vi "Write Type.vi"(8 "error in (no error)":errorcluster, 10 "Type":string, 11 "IV_data in":refnum<class "IV_data.lvclass">) -> (0 "error out":errorcluster, 3 "IV_data out":refnum<class "IV_data.lvclass">)   [LabVIEW 2018, in "IV_data.lvclass"]
uses:
  IV_data.lvclass
  Abstract/Data/Data2D/Data2D.lvclass
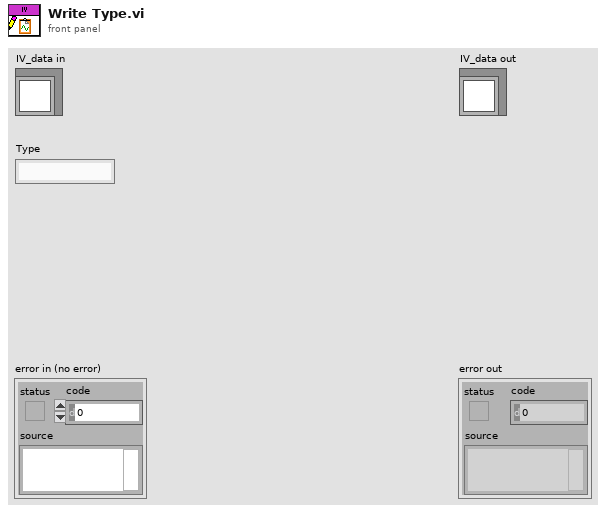
[diagram p1: front panel]
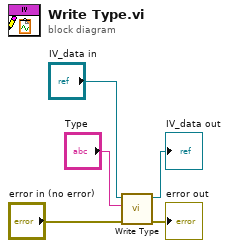
[diagram p0: block diagram]
diagram:
  n1 = call-parent "Write Type.vi"("error in (no error)"="error in (no error)", "Type"="Type", "Data2D in"="IV_data in") -> ("error out"=→"error out":errorcluster, "Data2D out"=→"IV_data out":refnum<class "IV_data.lvclass">)  [unwired: 7 in]
